vi "Decrypt dSpace.vi"(11 "Numeric in":u32) -> (1 "Lenkstatus":bool, 2 "wurde eingegriffen?":bool, 3 "Numeric out":u32)   [LabVIEW 2016]
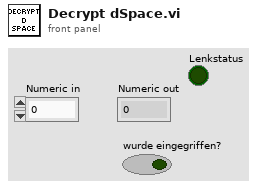
[diagram p1: front panel]
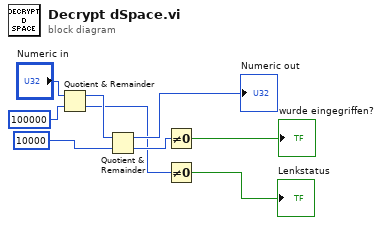
[diagram p0: block diagram]
diagram:
  n1 = Quotient & Remainder(x="Numeric in", y=u32 100000) -> (x-y*floor(x/y)=w3:u32, floor(x/y)=w2:u32)
  n2 = Quotient & Remainder(x=w3, y=u32 10000) -> (x-y*floor(x/y)=→"Numeric out":u32, floor(x/y)=w6:u32)
  n3 = Not Equal To 0?(x=w6) -> (x != 0?=→"wurde eingegriffen?":bool)
  n4 = Not Equal To 0?(x=w2) -> (x != 0?=→"Lenkstatus":bool)
